vi "TLB Native Dynamic Events ver 0.03.vi"() -> ()   [LabVIEW 2018]
uses:
  Labview Training Phase 2/Enum Controls/States for Action Engine.ctl
panel:
  out "QUEUE OUTPUT":string
  in  "Stop Queue":bool
  in  "Start Queue":bool
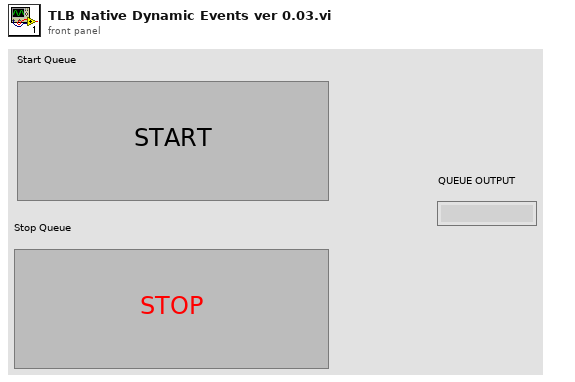
[diagram p1: front panel]
types:
  T1 = typedef "States for Action Engine.ctl" = enum16{"Initialize", "Write", "Read"}
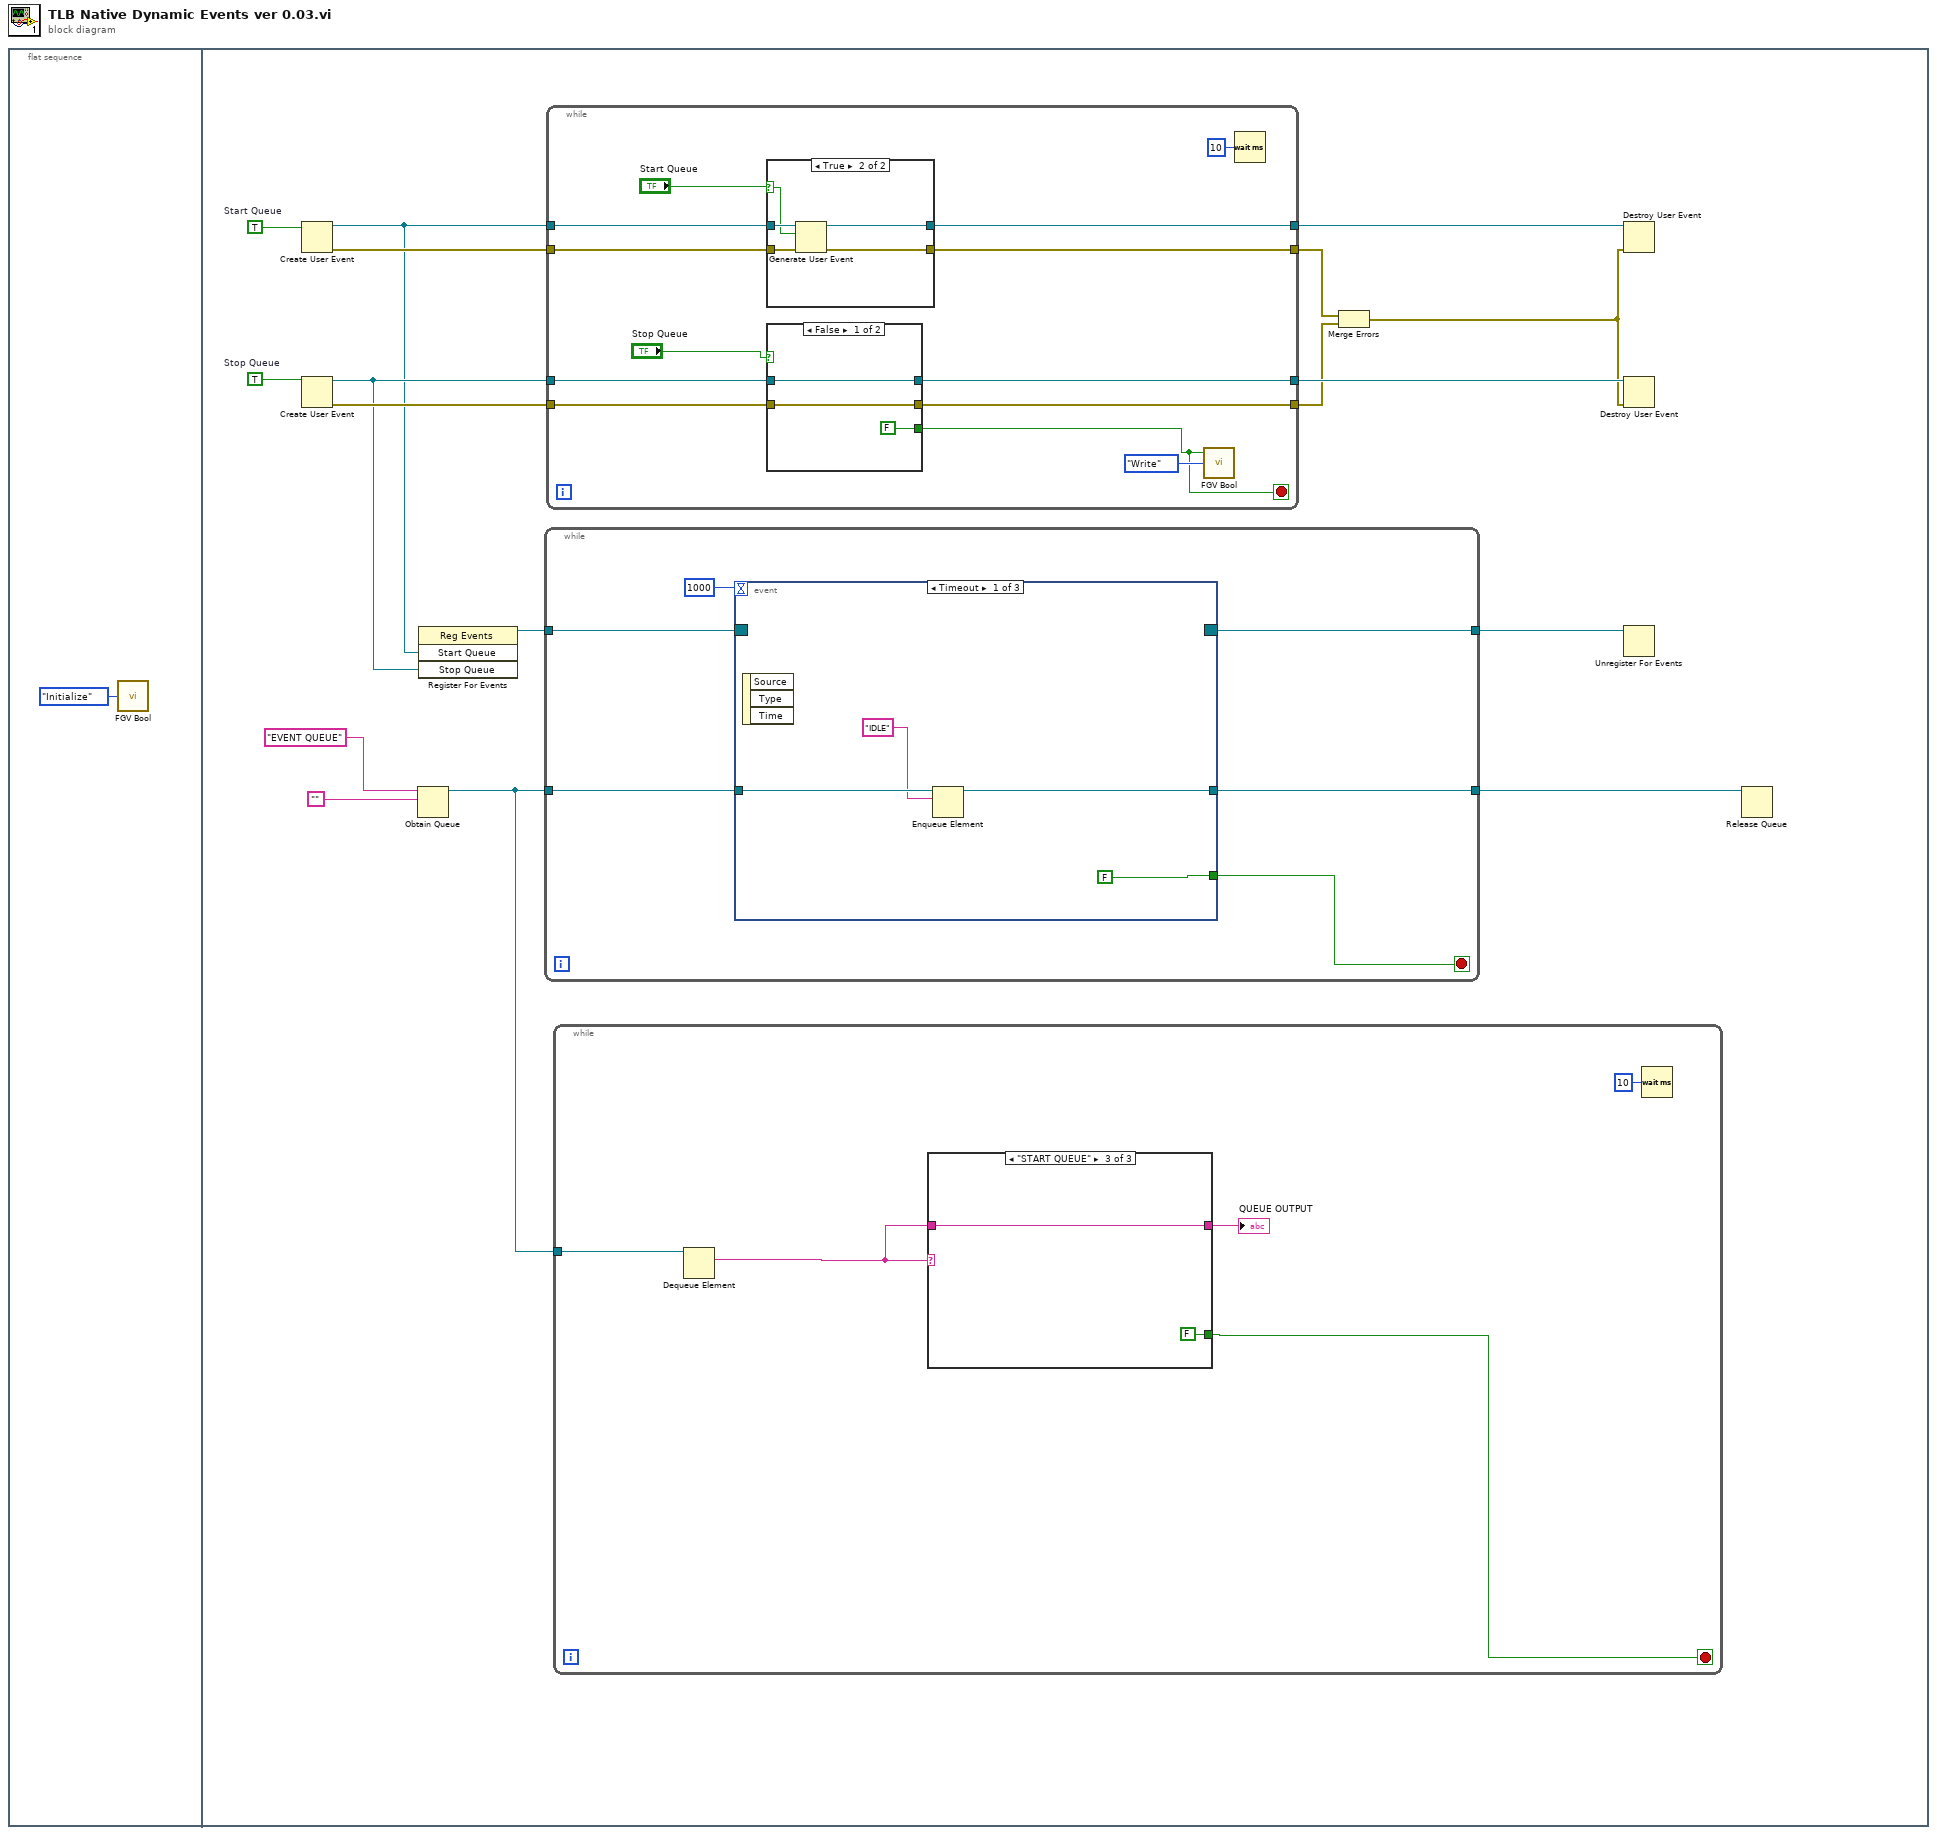
[diagram p0: block diagram]
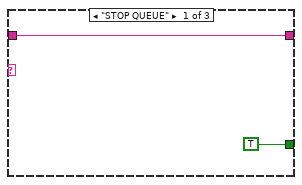
[diagram p2: hidden frame]
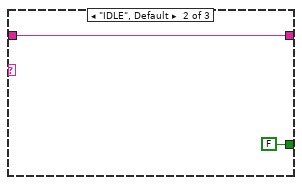
[diagram p3: hidden frame]
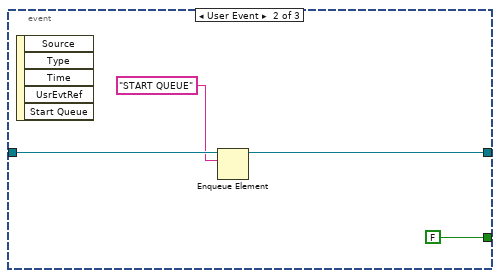
[diagram p4: hidden frame]
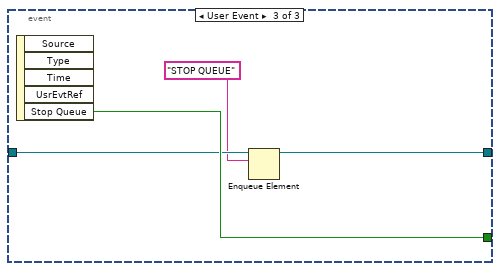
[diagram p5: hidden frame]
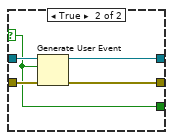
[diagram p6: hidden frame]
diagram:
  n1 = flat-sequence {
    frame #0 {
      n2 = call "FGV Bool.vi"("Init/Read/Write State"=States_for_Action_Engine."Initialize") -> ()  [unwired: 2 in, 2 out]
    }
    frame #1 {
      w18 = TRUE  # Stop Queue
      w17 = TRUE  # Start Queue
      n3 = Create User Event(user event datatype=w17) -> (user event=w8:refnum<user-event>, error out=w14:errorcluster)  [unwired: 1 in]
      n4 = Create User Event(user event datatype=w18) -> (user event=w9:refnum<user-event>, error out=w13:errorcluster)  [unwired: 1 in]
      n5 = Obtain Queue(name (unnamed)="EVENT QUEUE", element data type="") -> (queue out=w2:refnum<queue>)  [unwired: 3 in, 2 out]
      n6 = register-events(w8, w9) -> (reference out=w7:refnum<event-registration>)  [unwired: 2 in, 1 out]
      n7 = while {
        tunnel: w7 -> [w35]
        tunnel: [w34] -> w6
        tunnel: w2 -> [w32]
        tunnel: [w31] -> w5
        stop <- w33 stop-if-true
        n8 = event shown="[0] Timeout" {
          selector: w35 -> [_ _ _]
          dyn-events: [_ _ _] -> w34
          timeout: 1000 -> [_ _ _]
          tunnel: [FALSE FALSE w47] -> w33
          tunnel: w32 -> [w38 w42 w45]
          tunnel: [w37 w41 w46] -> w31
          event Timeout {
            n9 = event-data() -> ()  [unwired: 1 in, 3 out]
            n10 = Enqueue Element(queue=w38, element="IDLE") -> (queue out=w37:refnum<queue>)  [unwired: 2 in, 2 out]
          }
          event User Event {
            n11 = event-data() -> ()  [unwired: 1 in, 5 out]
            n12 = Enqueue Element(queue=w42, element="START QUEUE" ("name (unnamed)")) -> (queue out=w41:refnum<queue>)  [unwired: 2 in, 2 out]
          }
          event User Event {
            n13 = event-data() -> ("Stop Queue"=w47:bool)  [unwired: 1 in, 4 out]
            n14 = Enqueue Element(queue=w45, element="STOP QUEUE") -> (queue out=w46:refnum<queue>)  [unwired: 2 in, 2 out]
          }
        }
      }
      n15 = while {
        tunnel: w8 -> [w59]
        tunnel: w9 -> [w58]
        tunnel: [w57] -> w16
        tunnel: [w56] -> w15
        tunnel: w14 -> [w55]
        tunnel: [w54] -> w12
        tunnel: w13 -> [w53]
        tunnel: [w52] -> w11
        stop <- w48 stop-if-true
        n16 = case shown="True" "Start Queue" {
          selector: "Start Queue" -> [_ w71]
          tunnel: w59 -> [w70 w75]
          tunnel: [w70 w74] -> w56
          tunnel: w55 -> [w69 w73]
          tunnel: [w69 w72] -> w54
          frame False {
          }
          frame True {
            n17 = Generate User Event(user event=w75, event data cluster=w71, error in=w73) -> (user event out=w74:refnum<user-event>, error out=w72:errorcluster)  [unwired: 1 in]
          }
        }
        n18 = case shown="False" "Stop Queue" {
          selector: "Stop Queue" -> [_ w64]
          tunnel: w58 -> [w63 w68]
          tunnel: [w63 w67] -> w57
          tunnel: w53 -> [w62 w66]
          tunnel: [w62 w65] -> w52
          tunnel: [FALSE w64] -> w48
          frame False {
          }
          frame True {
            n19 = Generate User Event(user event=w68, event data cluster=w64, error in=w66) -> (user event out=w67:refnum<user-event>, error out=w65:errorcluster)  [unwired: 1 in]
          }
        }
        n20 = call "FGV Bool.vi"("Init/Read/Write State"=States_for_Action_Engine."Write", "Input Node"=w48) -> ()  [unwired: 1 in, 2 out]
        n21 = Wait (ms)(milliseconds to wait=u32 10) -> ()  [unwired: 1 out]
      }
      n22 = while {
        tunnel: w2 -> [w23]
        stop <- w19 stop-if-true
        n23 = Dequeue Element(queue=w23) -> (element=w22:string)  [unwired: 2 in, 3 out]
        n24 = case shown="\"START QUEUE\"" w22 {
          tunnel: w22 -> [w25 w27 w29]
          tunnel: [w25 w27 w29] -> w21
          tunnel: [TRUE FALSE FALSE] -> w19
          frame "STOP QUEUE" {
          }
          frame "IDLE", Default {
          }
          frame "START QUEUE" {
          }
        }
        "QUEUE OUTPUT" <- w21
        n25 = Wait (ms)(milliseconds to wait=u32 10) -> ()  [unwired: 1 out]
      }
      n26 = Merge Errors(w12, w11) -> (w10:errorcluster)
      n27 = Destroy User Event(user event=w15, error in=w10) -> ()  [unwired: 1 out]
      n28 = Destroy User Event(user event=w16, error in=w10) -> ()  [unwired: 1 out]
      n29 = Unregister For Events(event registration refnum=w6) -> ()  [unwired: 1 in, 1 out]
      n30 = Release Queue(queue=w5) -> ()  [unwired: 2 in, 3 out]
    }
  }
